vi "Create Trigger Model Digitize Block.vi"(8 "error in (no error)":errorcluster, 9 "Buffer Name (defbuffer1)":string, 11 "VISA resource name":refnum<visa-resource-name>) -> (0 "error out":errorcluster, 3 "VISA resource name out":refnum<visa-resource-name>)   [LabVIEW 2009, in "Keithley DMM7510.lvlib"]
doc: "This VI defines a trigger block that makes a digitize measurement."
uses:
  Keithley DMM7510.lvlib
panel:
  in  "Count":i16
  in  "Block Number (1)":i32 min=1 format="%#.6g"
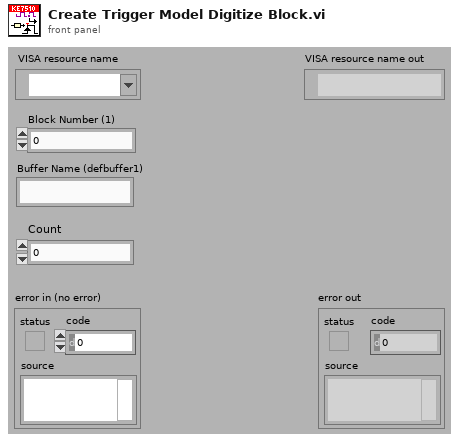
[diagram p1: front panel]
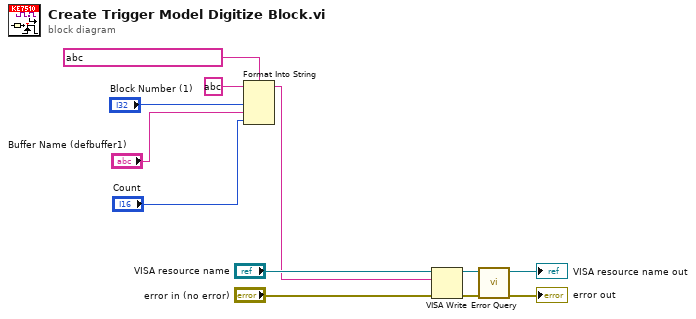
[diagram p0: block diagram]
diagram:
  n1 = Format Into String(format string=string ?, initial string=string ?, "Block Number (1)", "Buffer Name (defbuffer1)", "Count") -> (resulting string=w3:string)  [unwired: 1 in, 1 out]
  n2 = VISA Write(VISA resource name="VISA resource name", write buffer=w3, error in (no error)="error in (no error)") -> (VISA resource name out=w8:refnum<visa-resource-name>, error out=w7:errorcluster)  [unwired: 1 out]
  n3 = call "Error Query.vi"("error in (no error)"=w7, "VISA resource name"=w8) -> ("error out"=→"error out":errorcluster, "VISA resource name out"=→"VISA resource name out":refnum<visa-resource-name>)  [unwired: 8 out]
